vi "StartMeas.vi"(8 "error in (no error)":errorcluster, 11 "NhRegenGridSim in":refnum<class "NhRegenGridSim.lvclass">) -> (0 "error out":errorcluster, 3 "NhRegenGridSim out":refnum<class "NhRegenGridSim.lvclass">)   [LabVIEW 2018, in "AcPwrPlugins.lvlib" / "NhRegenGridSim.lvclass"]
uses:
  NhRegenGridSim.lvclass
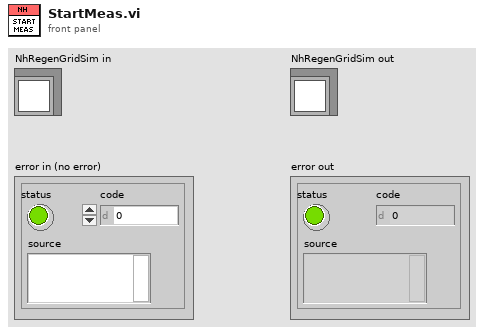
[diagram p1: front panel]
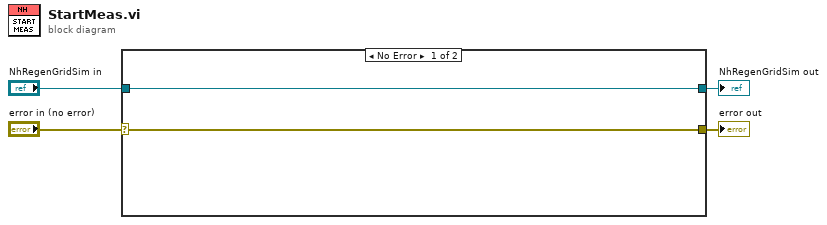
[diagram p0: block diagram]
diagram:
  n1 = case shown="No Error" "error in (no error)" {
    selector: "error in (no error)" -> [w5 w7]
    tunnel: [w5 w7] -> w4
    tunnel: [w6 w8] -> w3
    tunnel: "NhRegenGridSim in" -> [w6 w8]
    frame No Error {
    }
    frame Error {
    }
  }
  "error out" <- w4
  "NhRegenGridSim out" <- w3
